vi "flag experiment state.vi"(8 "error in (no error)":errorcluster, 9 "filename":string="CS_EtAc_SLi_0to50_20_10min_habituation_201301051650", 10 "data directory":path=path "B:/lady gaga/olfaction/EtAc Spatial Linear 0 to 50 ppm 20 cm 10min_habituation/CS/20130105/1650", 11 "experiment started":bool) -> (0 "error out":errorcluster)   [LabVIEW 2021]
uses:
  experiment state global.vi
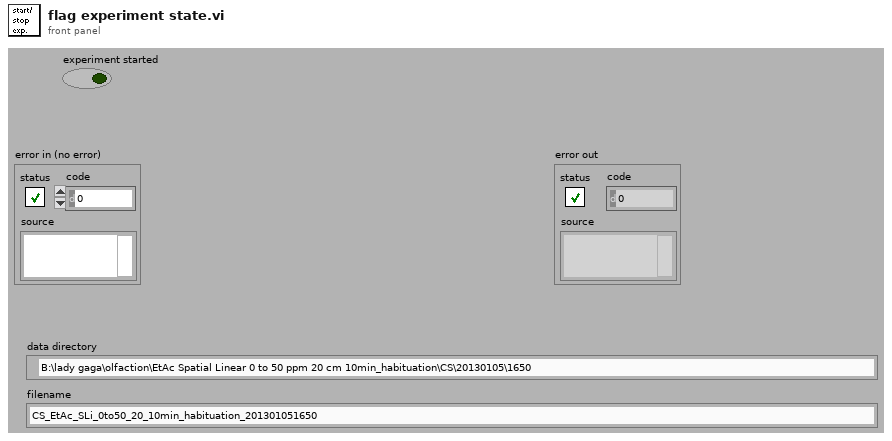
[diagram p1: front panel]
types:
  T1 = cluster{"experiment started":bool, "experiment ended":bool, "experiment start time":u32}
  T2 = cluster{"data directory":path, "filename":string}
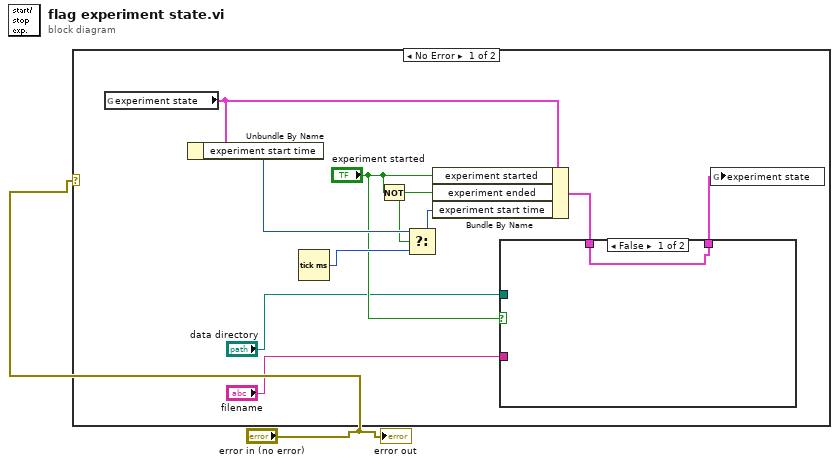
[diagram p0: block diagram]
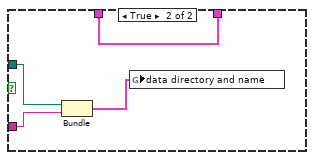
[diagram p2: hidden frame]
diagram:
  n1 = case shown="No Error" "error in (no error)" {
    frame No Error {
      n2 = global read "experiment state global.vi" "experiment state"() -> (w10:T1)
      n3 = Unbundle By Name(w10) -> ("experiment start time"=w9:u32)
      n4 = Tick Count (ms)() -> (millisecond timer value=w7:u32)
      n5 = Not(x="experiment started") -> (.not. x?=w8:bool)
      n6 = Select(t=w9, s=w8, f=w7) -> (s? t:f=w11:u32)
      n7 = Bundle By Name(cluster=w10, "experiment started"="experiment started", "experiment ended"=w8, "experiment start time"=w11) -> (w3:T1)
      n8 = case shown="False" "experiment started" {
        tunnel: "data directory" -> [_ w16]
        tunnel: "filename" -> [_ w15]
        tunnel: w3 -> [w12 w13]
        tunnel: [w12 w13] -> w2
        frame False {
        }
        frame True {
          n9 = Bundle("data directory"=w16, "filename"=w15) -> (w14:T2)  [unwired: 1 in]
          n10 = global write "experiment state global.vi" "data directory and name"(w14) -> ()
        }
      }
      n11 = global write "experiment state global.vi" "experiment state"(w2) -> ()
    }
    frame Error {
    }
  }
  "error out" <- "error in (no error)"
